vi "TrEqSolver.vi"(9 "D":dbl, 10 "B":dbl, 11 "A":dbl) -> (1 "Solution Exists":bool, 2 "angle 2":dbl, 3 "angle 1":dbl)   [LabVIEW 2017, in "NI_Robotics_AnalyticKinematics.lvlib"]
uses:
  <vilib>/robotics/Kinematics/Analytical/NI_Robotics_AnalyticKinematics.lvlib
panel:
  # "Solve Acos(angle)+Bsin(angle) +D =0"
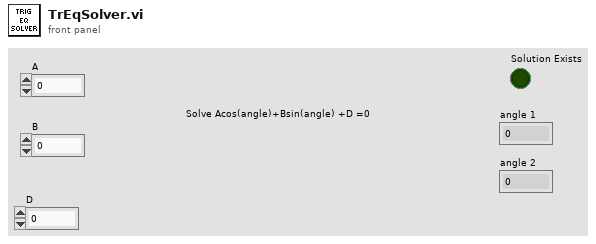
[diagram p1: front panel]
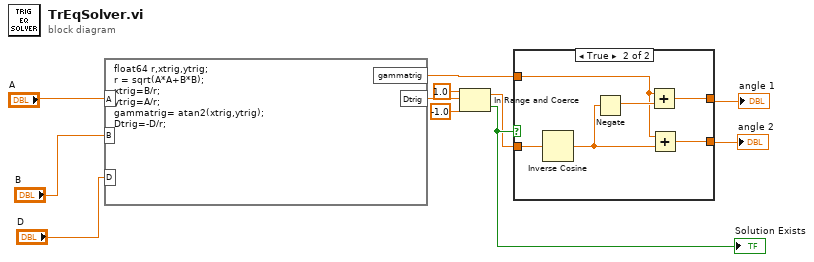
[diagram p0: block diagram]
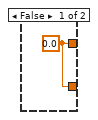
[diagram p2: hidden frame]
diagram:
  n1 = formula code="float64 r,xtrig,ytrig;\nr = sqrt(A*A+B*B);\nxtrig=B/r;\nytrig=A/r;\ngammatrig= atan2(xtrig,ytrig);\nDtrig=-D/r;"("A"="A", "B"="B", "D"="D") -> ("Dtrig"=w8:dbl, "gammatrig"=w3:dbl)
  n2 = In Range and Coerce(upper limit=1.0, x=w8, lower limit=-1.0) -> (coerced(x)=w4:dbl, In Range?=w5:bool)
  "Solution Exists" <- w5
  n3 = case shown="True" w5 {
    tunnel: w4 -> [_ w18]
    tunnel: w3 -> [_ w15]
    tunnel: [w12 w14] -> w1
    tunnel: [w12 w13] -> w2
    frame False {
      w12 = 0.0
    }
    frame True {
      n4 = Inverse Cosine(1:w18) -> (0:w17:dbl)
      n5 = Negate(x=w17) -> (-x=w16:dbl)
      n6 = Add(x=w15, y=w16) -> (x+y=w14:dbl)
      n7 = Add(x=w15, y=w17) -> (x+y=w13:dbl)
    }
  }
  "angle 1" <- w1
  "angle 2" <- w2
